vi "Create Reference.vi"(10 "uid":string, 11 "class":string) -> (3 "Reference":refnum<class "Reference.lvclass">)   [LabVIEW 2018, in "VILab.lvlib" / "Reference.lvclass"]
uses:
  Reference.lvclass
  C:/Users/Flarn/Documents/LabVIEW Projects/Low-Level VI Manipulation/Support Files/VILab/Element.lvclass
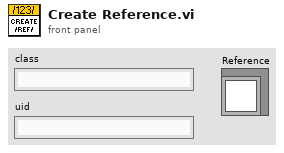
[diagram p1: front panel]
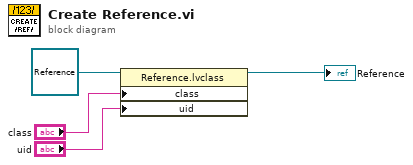
[diagram p0: block diagram]
diagram:
  n1 = property class="Reference.lvclass"(reference=refnum<class "Reference.lvclass"> refnum ("VILab.lvlib:Reference.lvclass"), "class"="class", "uid"="uid") -> (reference out=→"Reference":refnum<class "Reference.lvclass">)  [unwired: 1 in, 1 out]
